vi "Multichannel Recording0.2.vi"() -> ()   [LabVIEW 2014]
uses:
  Enum State Typedef.ctl
  <vilib>/Utility/error.llb/DialogType.ctl
  <vilib>/_DAQmxBase/Internals/DAQmxBase Create Channel (AI-Voltage-Basic).vi
  <vilib>/_DAQmxBase/Internals/DAQmxBase Timing (Sample Clock).vi
  <vilib>/_DAQmxBase/Internals/DAQmxBase Read (Analog 2D DBL NChan NSamp).vi
panel:
  in  "Open Button":bool
  in  "Tab Control":T1(tab)
  in  "Use Channel 0":bool caption="In Use?"
  in  "Amplifier Channel 0":T2 {"Amplifier Model" items=["Select a Model", "AM 1700", "BMA 200"]}
  out "Channel 0 Chart":waveform(dbl)(graph)
  in  "User Data Channel 0":T3
  in  "Use Channel 1":bool caption="In Use?"
  out "Channel 1 Chart":waveform(dbl)(graph)
  in  "User Data Channel 1":T3
  in  "Amplifier Channel 1":T2 {"Amplifier Model" items=["Select a Model", "AM 1700", "BMA 200"]}
  in  "Use Channel 2":bool caption="In Use?"
  out "Channel 2 Chart":waveform(dbl)(graph)
  in  "User Data Channel 2":T3
  in  "Amplifier Channel 2":T2 {"Amplifier Model" items=["Select a Model", "AM 1700", "BMA 200"]}
  in  "Use Channel 3":bool caption="In Use?"
  out "Channel 3 Chart":waveform(dbl)(graph)
  in  "User Data Channel 3":T3
  in  "Amplifier Channel 3":T2 {"Amplifier Model" items=["Select a Model", "AM 1700", "BMA 200"]}
  out "Overview Chart":waveform(dbl)[](graph)
  in  "Stop Preview":bool
  in  "OK Button":bool
  out "State":T4
  in  "Clear Display":bool
  in  "Preview Button":bool
  out "Iterations Recorded":i32
  in  "Recording Time (seconds)":dbl
  in  "Sample Rate":i32=1000
  in  "Stop Button":bool
  out "Start Time hr/min":string
  out "Date mm/dd/yy":string
  in  "Exit Button":bool
  in  "Record Button":bool
  # "MSU EFISH Lab Multi-Channel Electronic Pulse Recorder"
  # "Must enter numbers into here before you start"
  # "Blue for On\nOrange for Off"
  # "DC"
  # "AC"
  # "Blue for AC and Orange for DC"
  # "Blue for On\nOrange for Off"
  # "DC"
  # "AC"
  # "Blue for AC and Orange for DC"
  # "Blue for On\nOrange for Off"
  # "DC"
  # "AC"
  # "Blue for AC and Orange for DC"
  # "Blue for On\nOrange for Off"
  # "DC"
  # "AC"
  # "Blue for AC and Orange for DC"
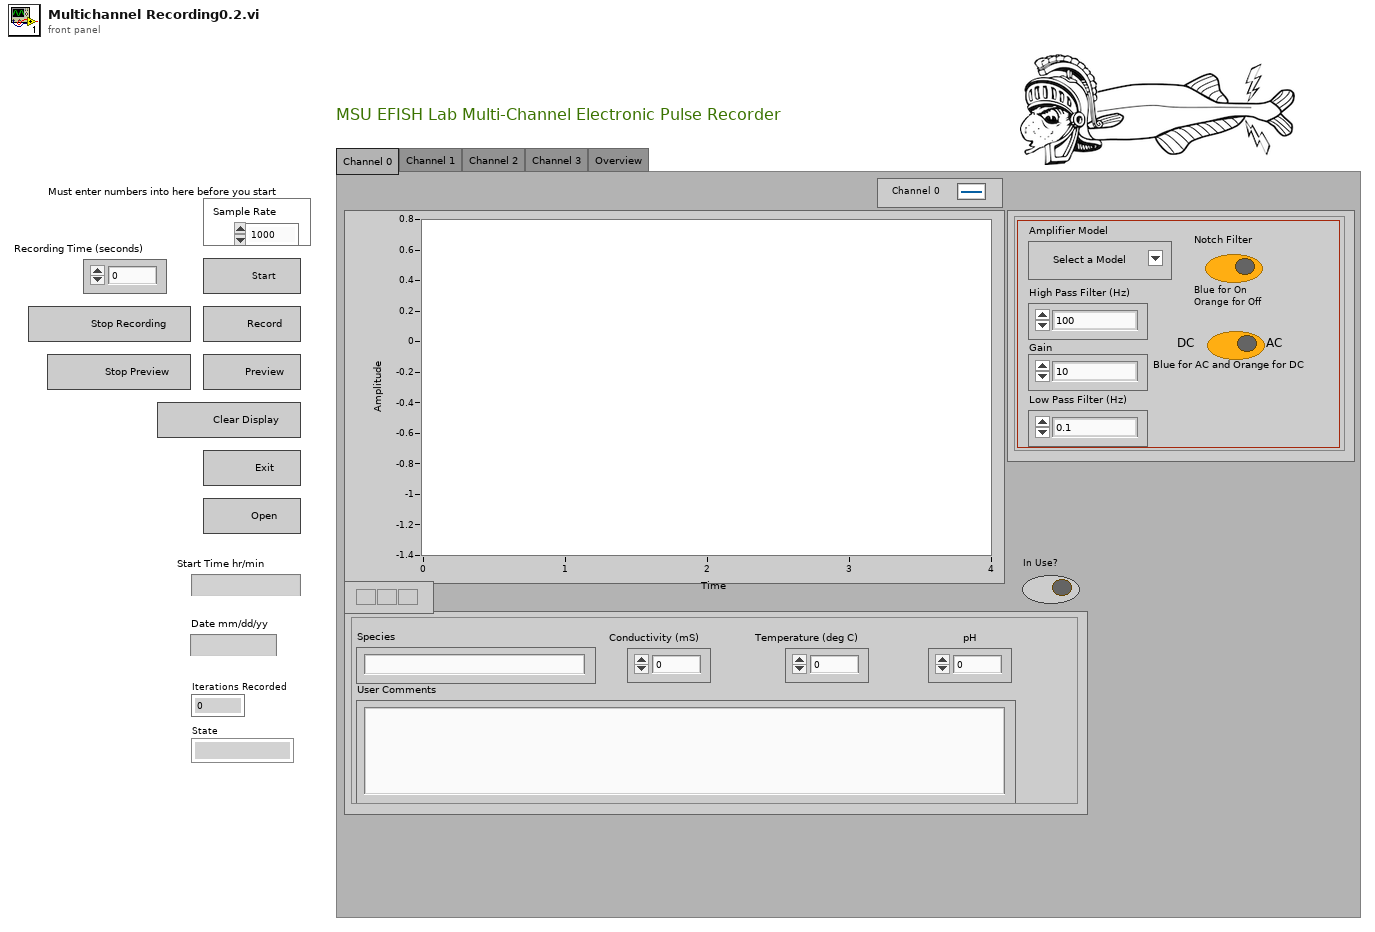
[diagram p1: front panel]
types:
  T1 = enum32{"Channel 0", "Channel 1", "Channel 2", "Channel 3", "Overview"}
  T2 = cluster{"Low Pass Filter (Hz)":enum16{"0.1", "1", "3", "10", "30", "100", "300"}, "Gain ":enum16{"10", "20", "50", "100", "200", "500", "1000", "2k", "5k", "10k", "20k", "50k"}, "High Pass Filter (Hz)":enum16{"100", "500", "1000", "3000", "5000", "10,000", "20,000", "30,000", "50,000"}, "Notch Filter":bool, "Amplifier Model":u16, "AC/DC Switch":bool}
  T3 = cluster{"pH":dbl, "Conductivity (mS)":dbl, "Temperature (deg C)":dbl, "User Comments":string, "Species":string}
  T4 = typedef "Enum State Typedef.ctl" = enum16{"", "Open FIle", "Beginning State", "Set the Sample Clock", "Prepreview Handling", "Clear Display", "Preview Data", "Stop", "Exit", "Record", "Create File"}
  T5 = enum16{"open", "open or create", "create or replace", "create", "open (read-only)"}
  T6 = cluster{"Waveform":waveform(dbl), "Waveform":waveform(dbl), "Waveform":waveform(dbl), "Waveform":waveform(dbl), waveform(dbl)[]}
  T7 = cluster{"tdms file out":refnum<k34>, "tdms file out":refnum<k34>, "tdms file out":refnum<k34>, "tdms file out":refnum<k34>}
  T8 = cluster{"Use Channel 0":bool, "Use Channel 1":bool, "Use Channel 2":bool, "Use Channel 3":bool}
  T9 = typedef "DialogType.ctl" = u16
  T10 = cluster{"data":dbl[][], dbl[][], i32, i32, dbl, "Use Channel 0":bool}
  T11 = cluster{"data":dbl[][], dbl[][], i32, i32, dbl, "Use Channel 1":bool}
  T12 = cluster{"data":dbl[][], dbl[][], i32, i32, dbl, "Use Channel 2":bool}
  T13 = cluster{"data":dbl[][], dbl[][], i32, i32, dbl, "Use Channel 3":bool}
  T14 = cluster{"Waveform":waveform(dbl), "Waveform":waveform(dbl), "Waveform":waveform(dbl), "Waveform":waveform(dbl)}
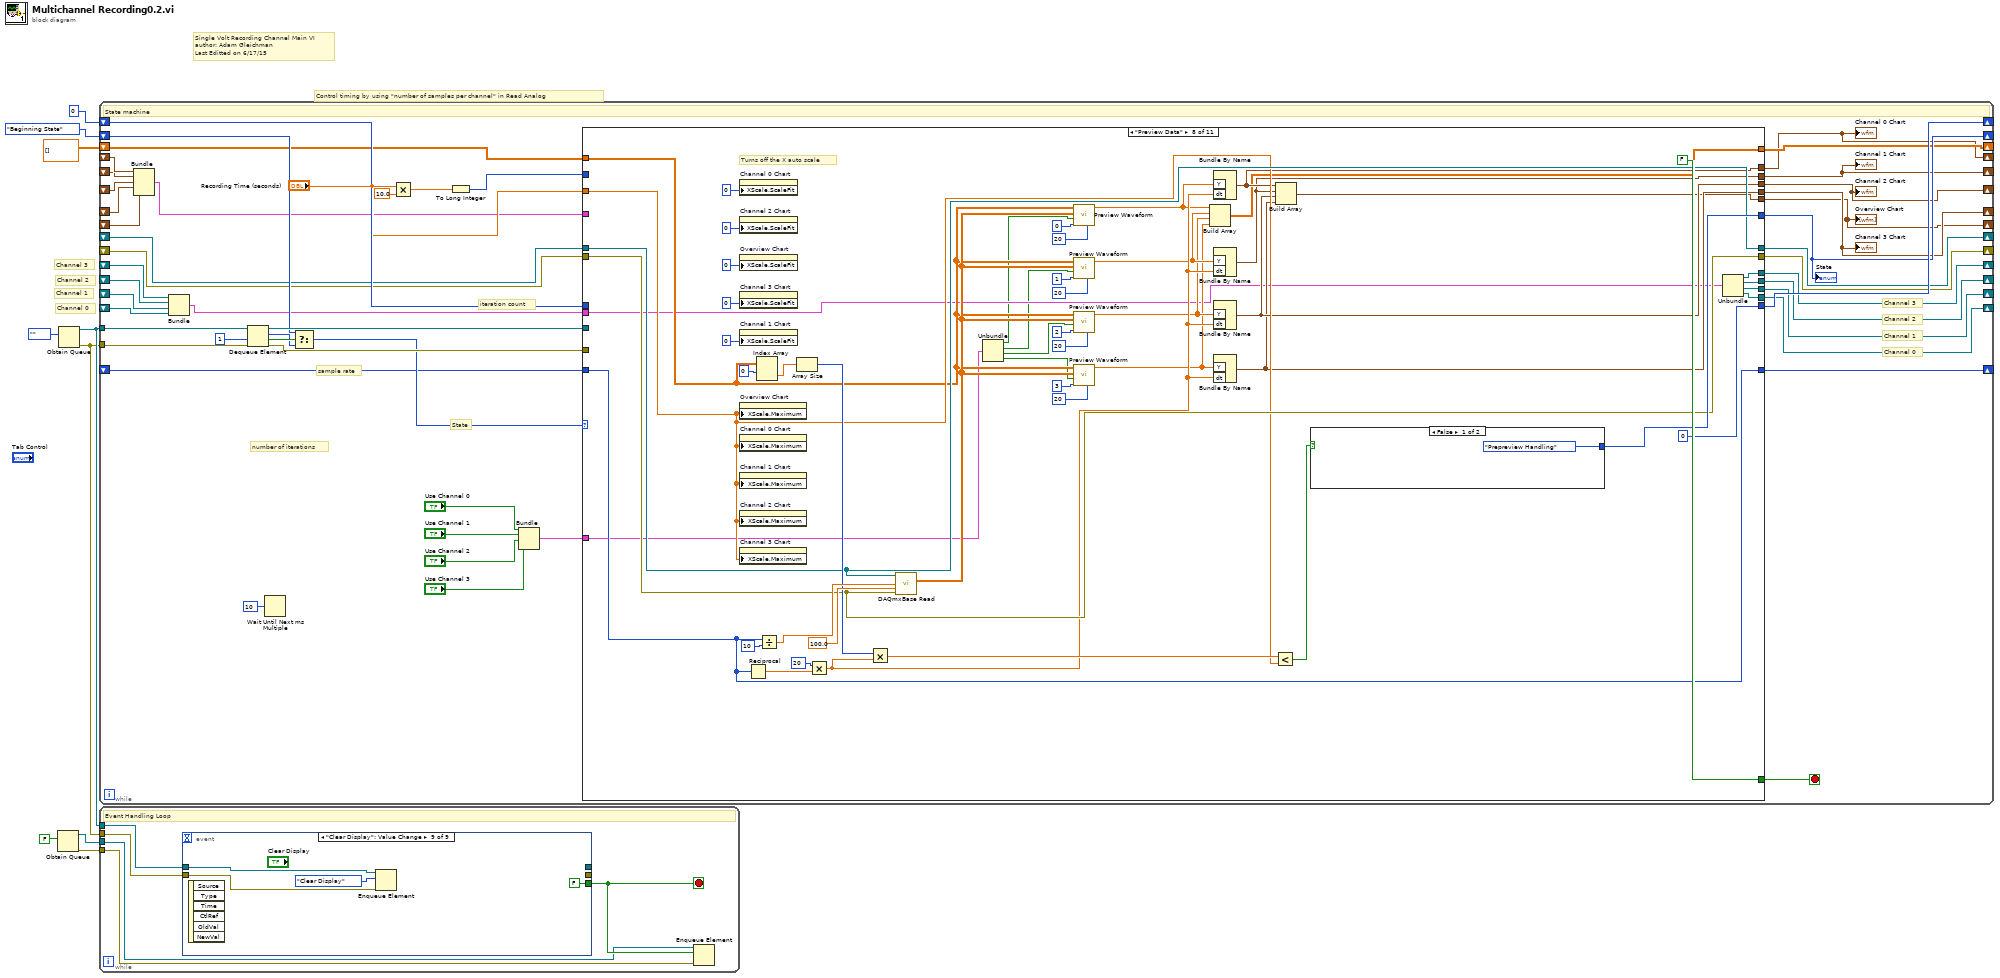
[diagram p0: block diagram]
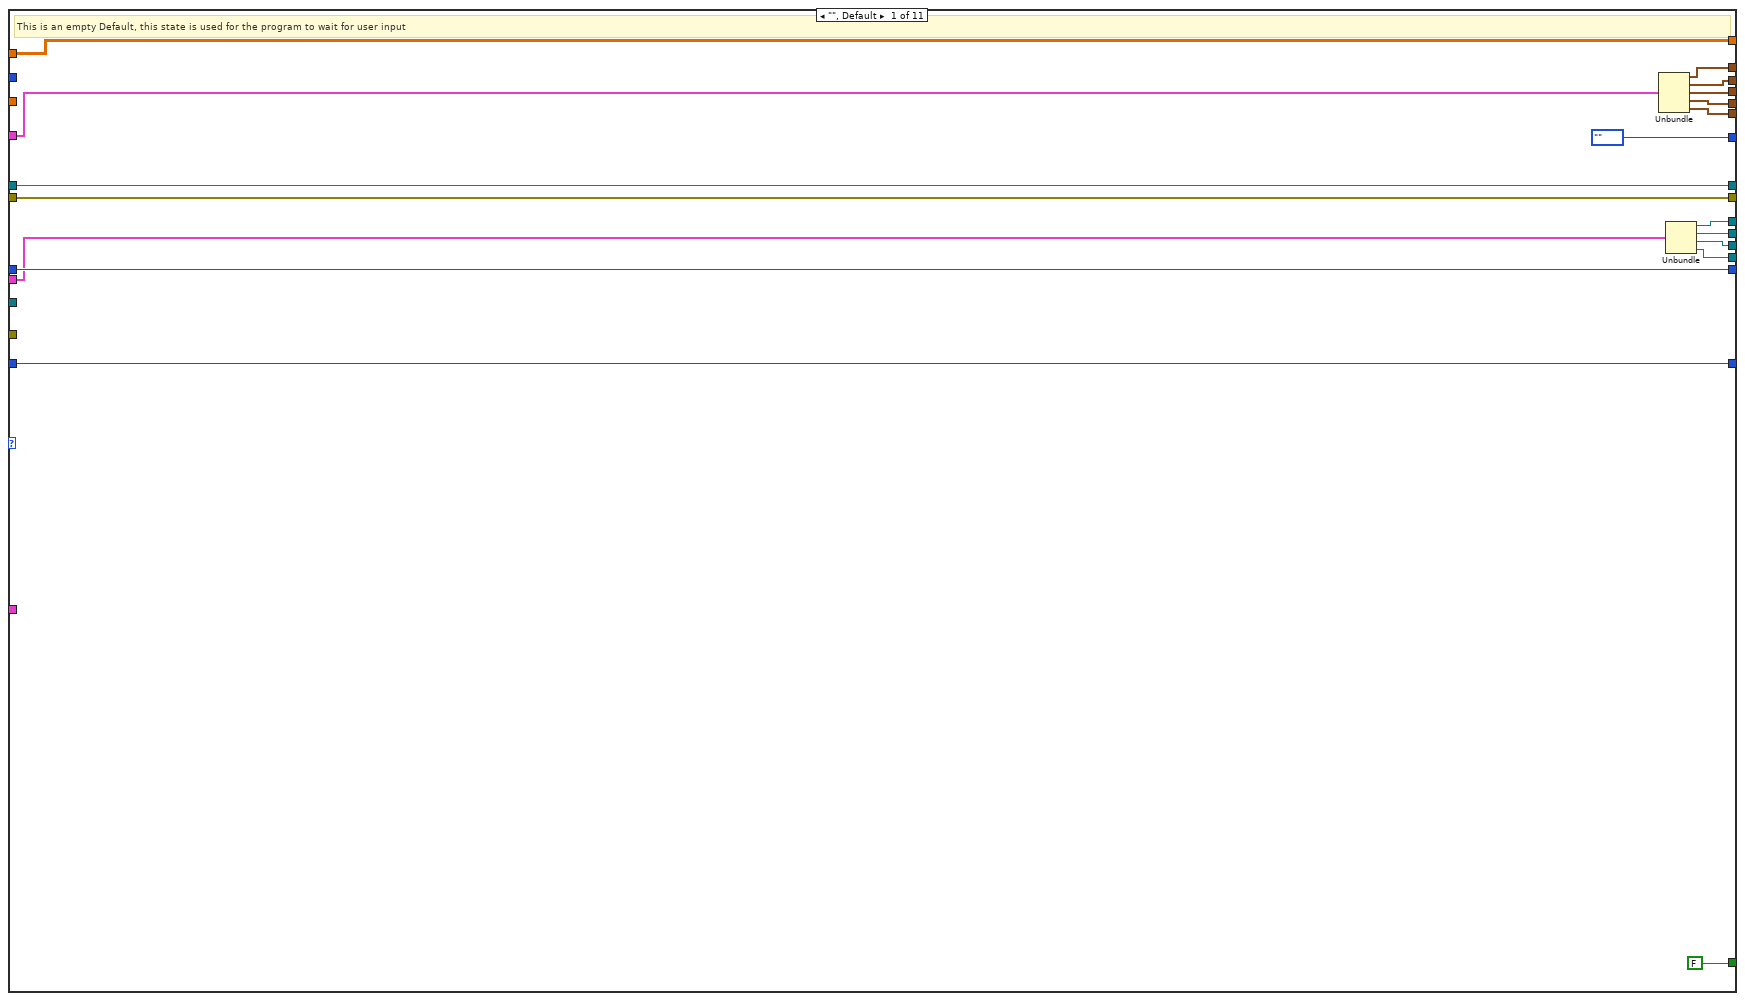
[diagram p2: hidden frame]
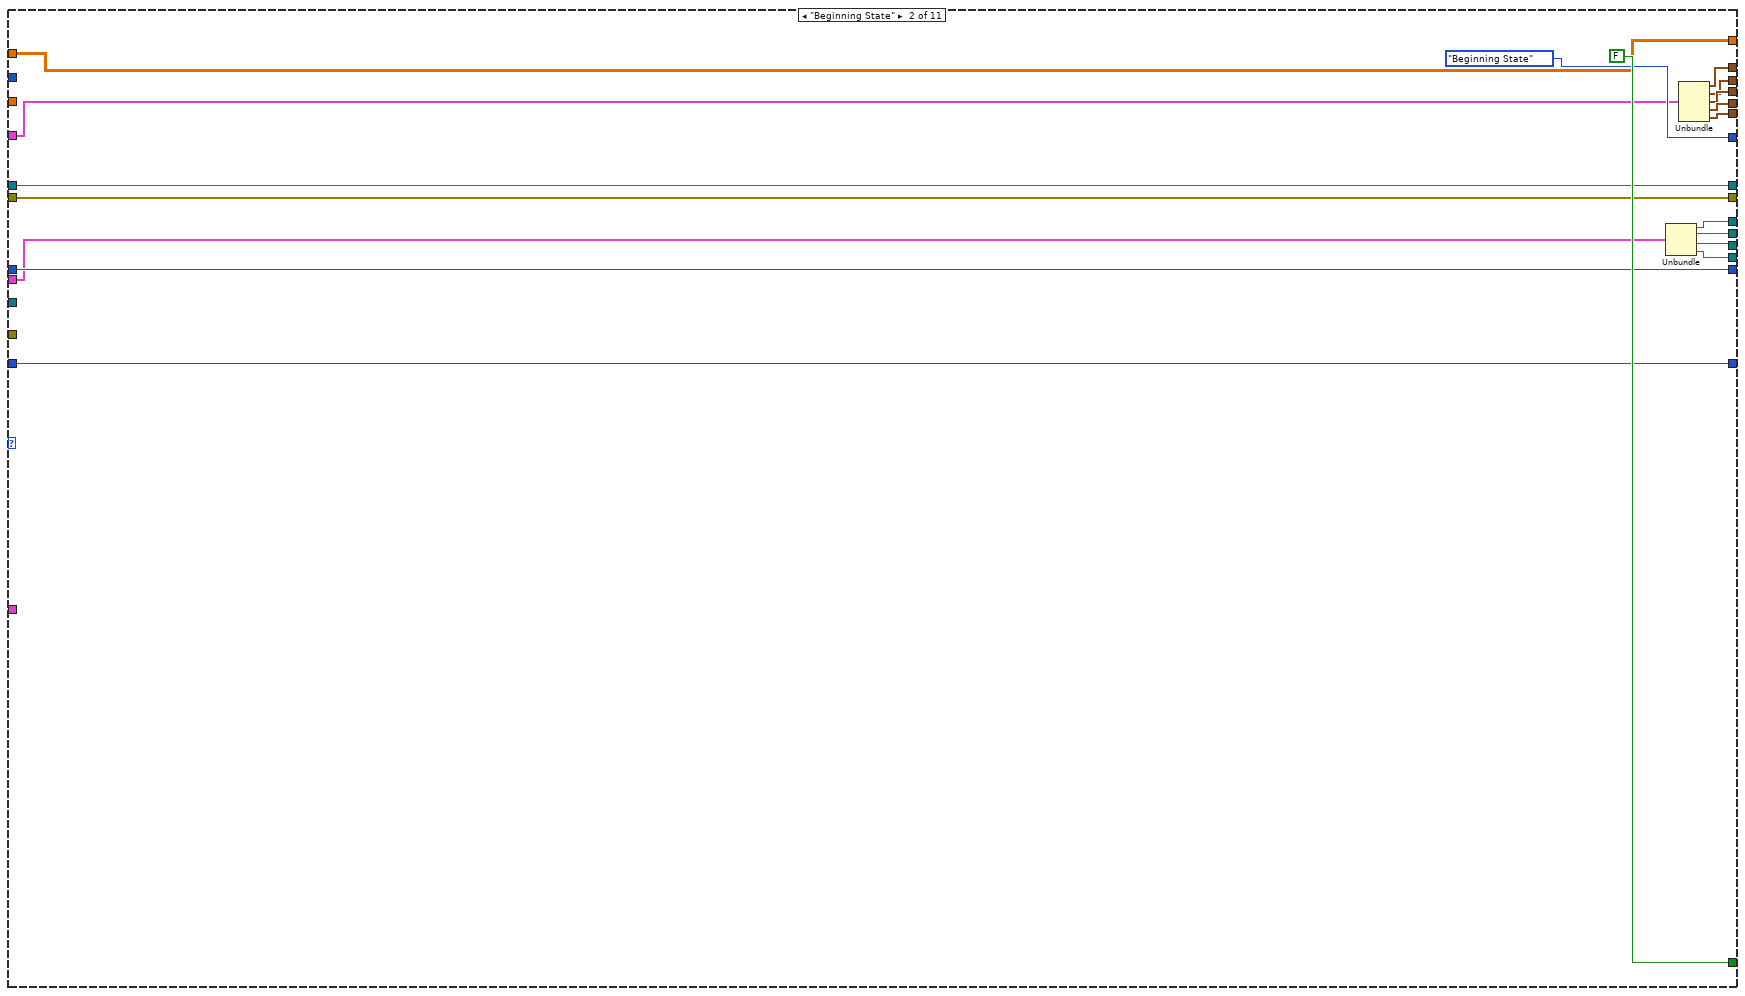
[diagram p3: hidden frame]
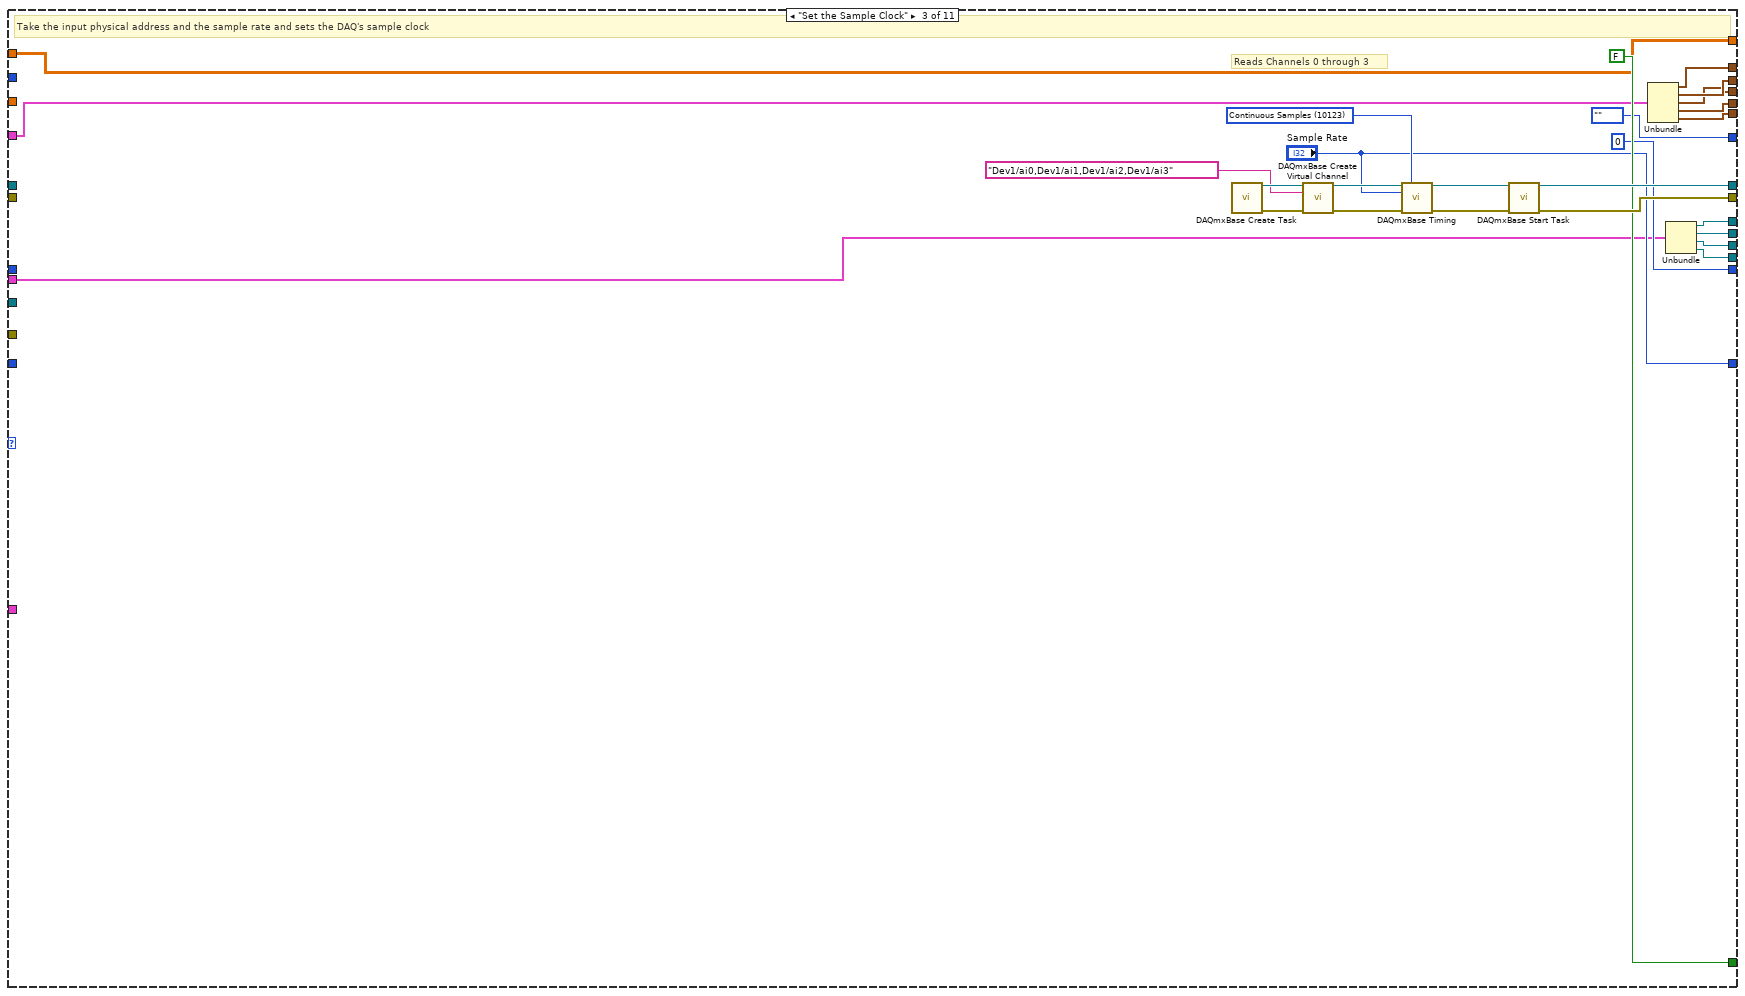
[diagram p4: hidden frame]
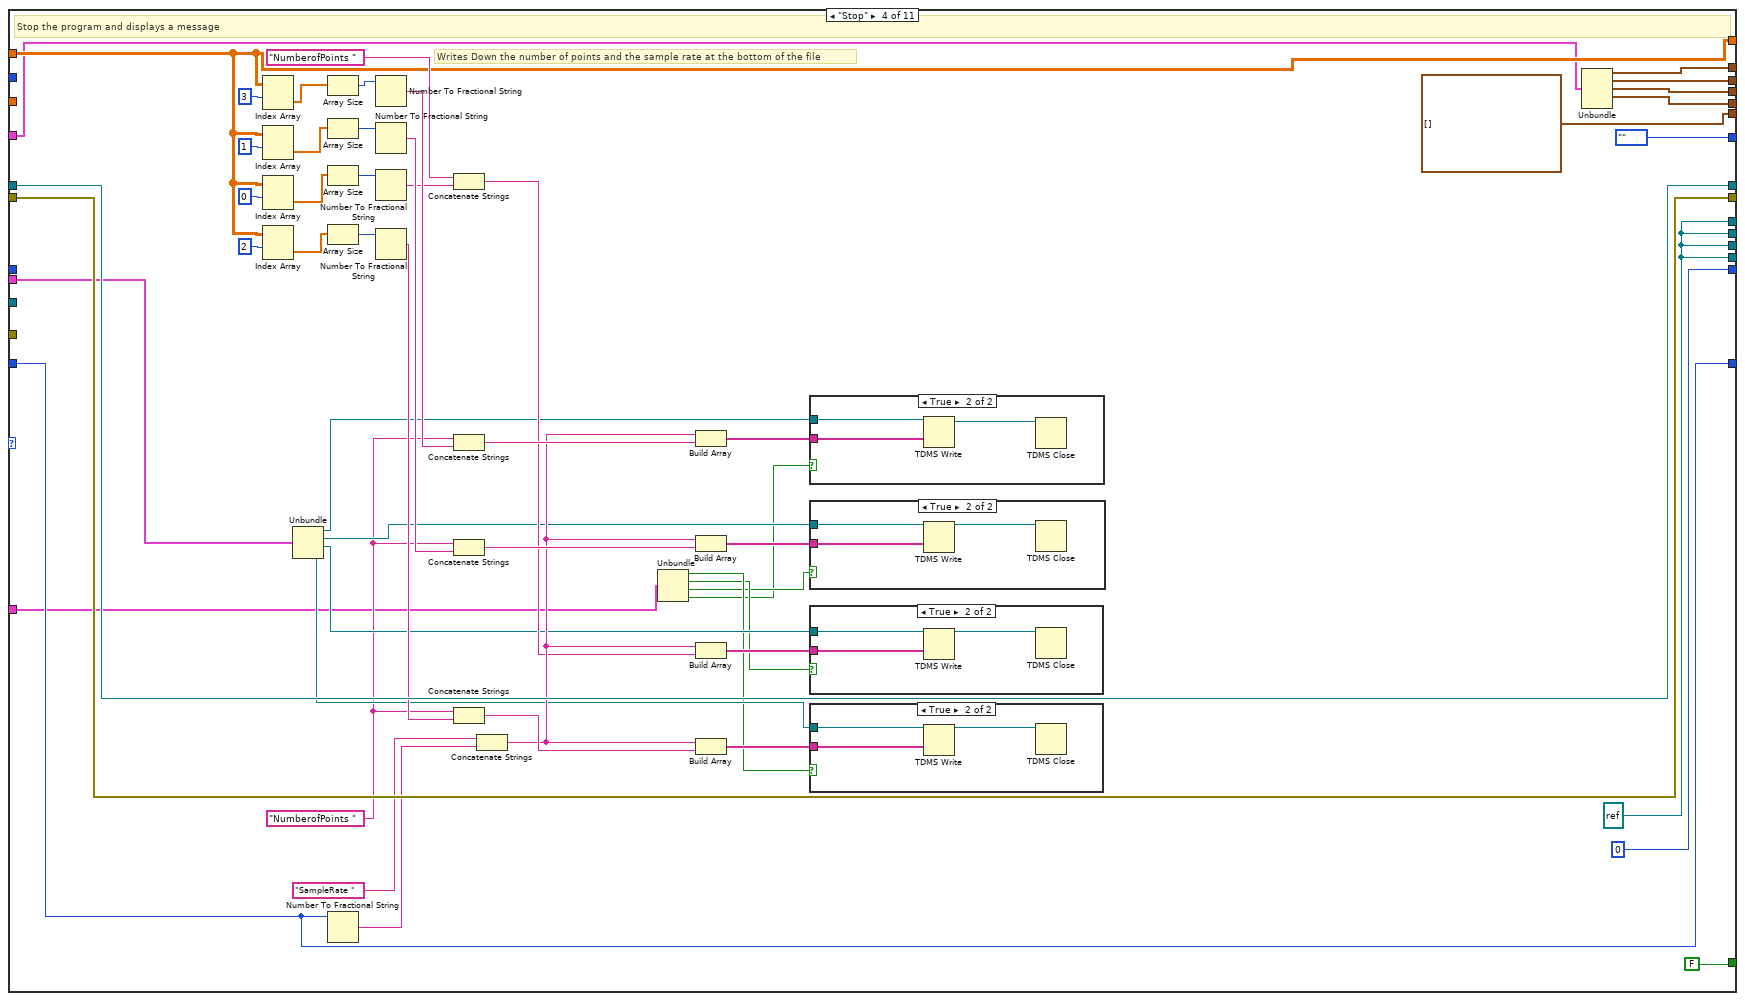
[diagram p5: hidden frame]
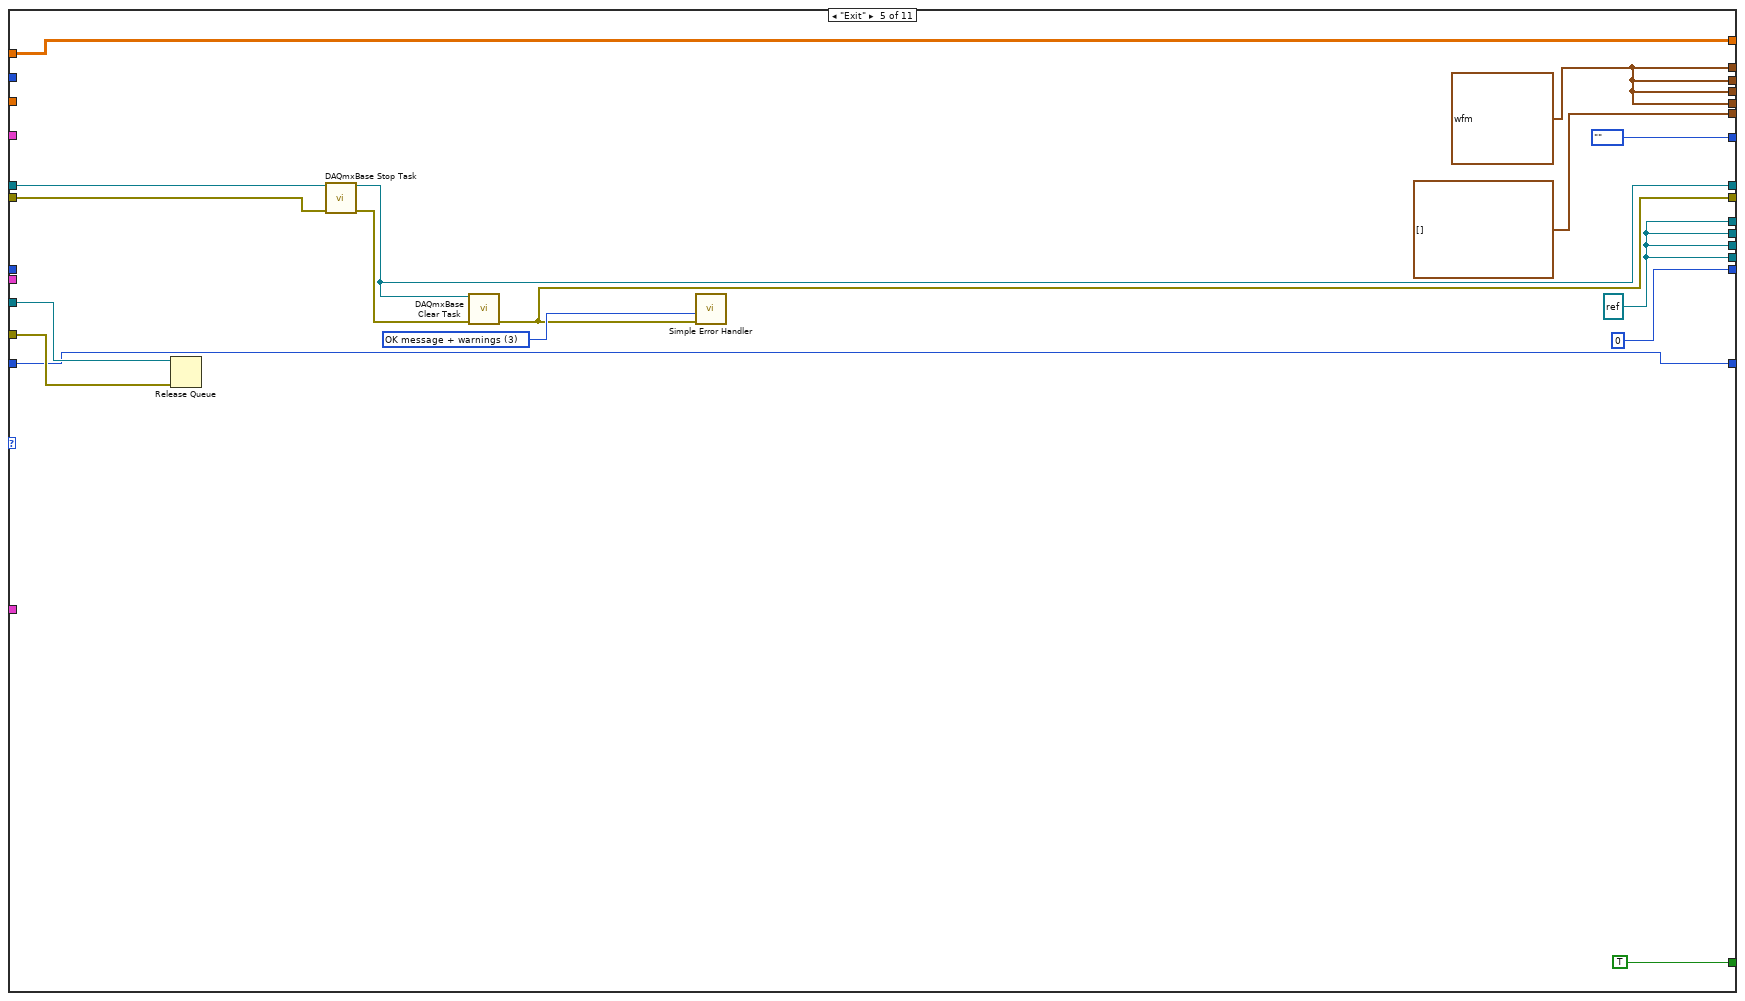
[diagram p10: hidden frame]
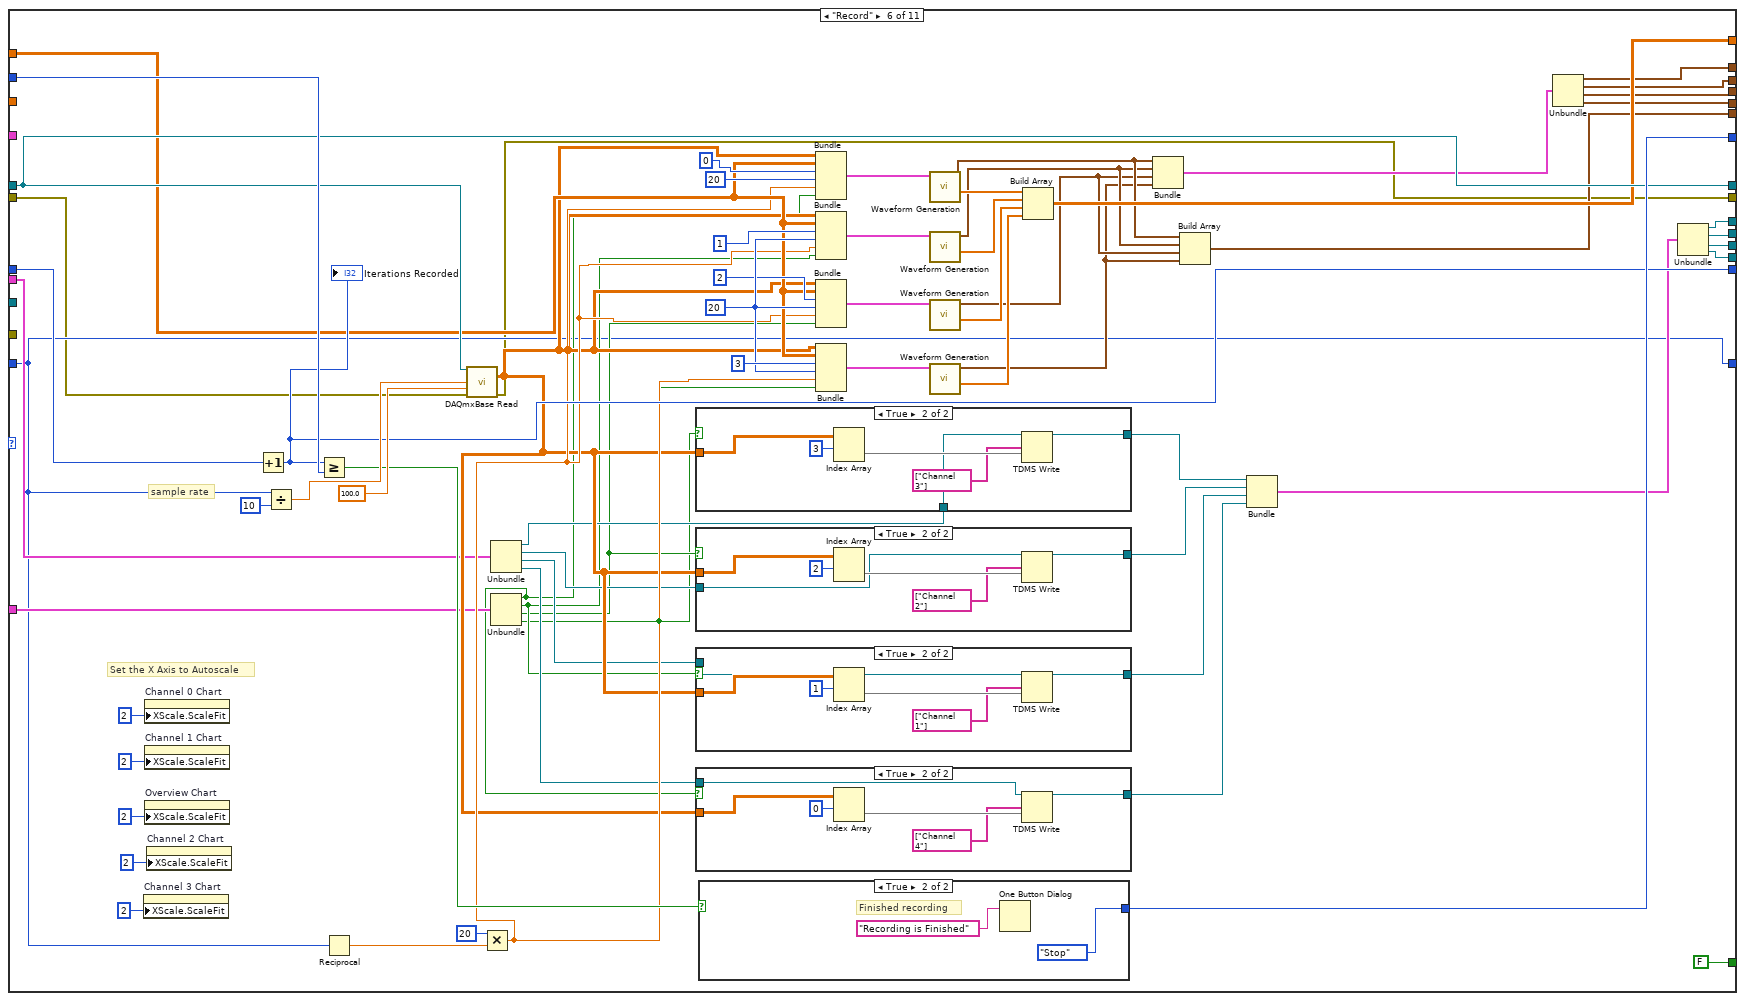
[diagram p11: hidden frame]
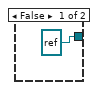
[diagram p12: hidden frame]
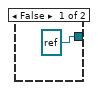
[diagram p13: hidden frame]
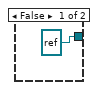
[diagram p14: hidden frame]
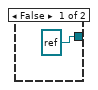
[diagram p15: hidden frame]
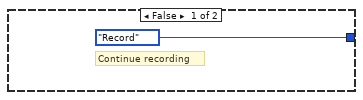
[diagram p16: hidden frame]
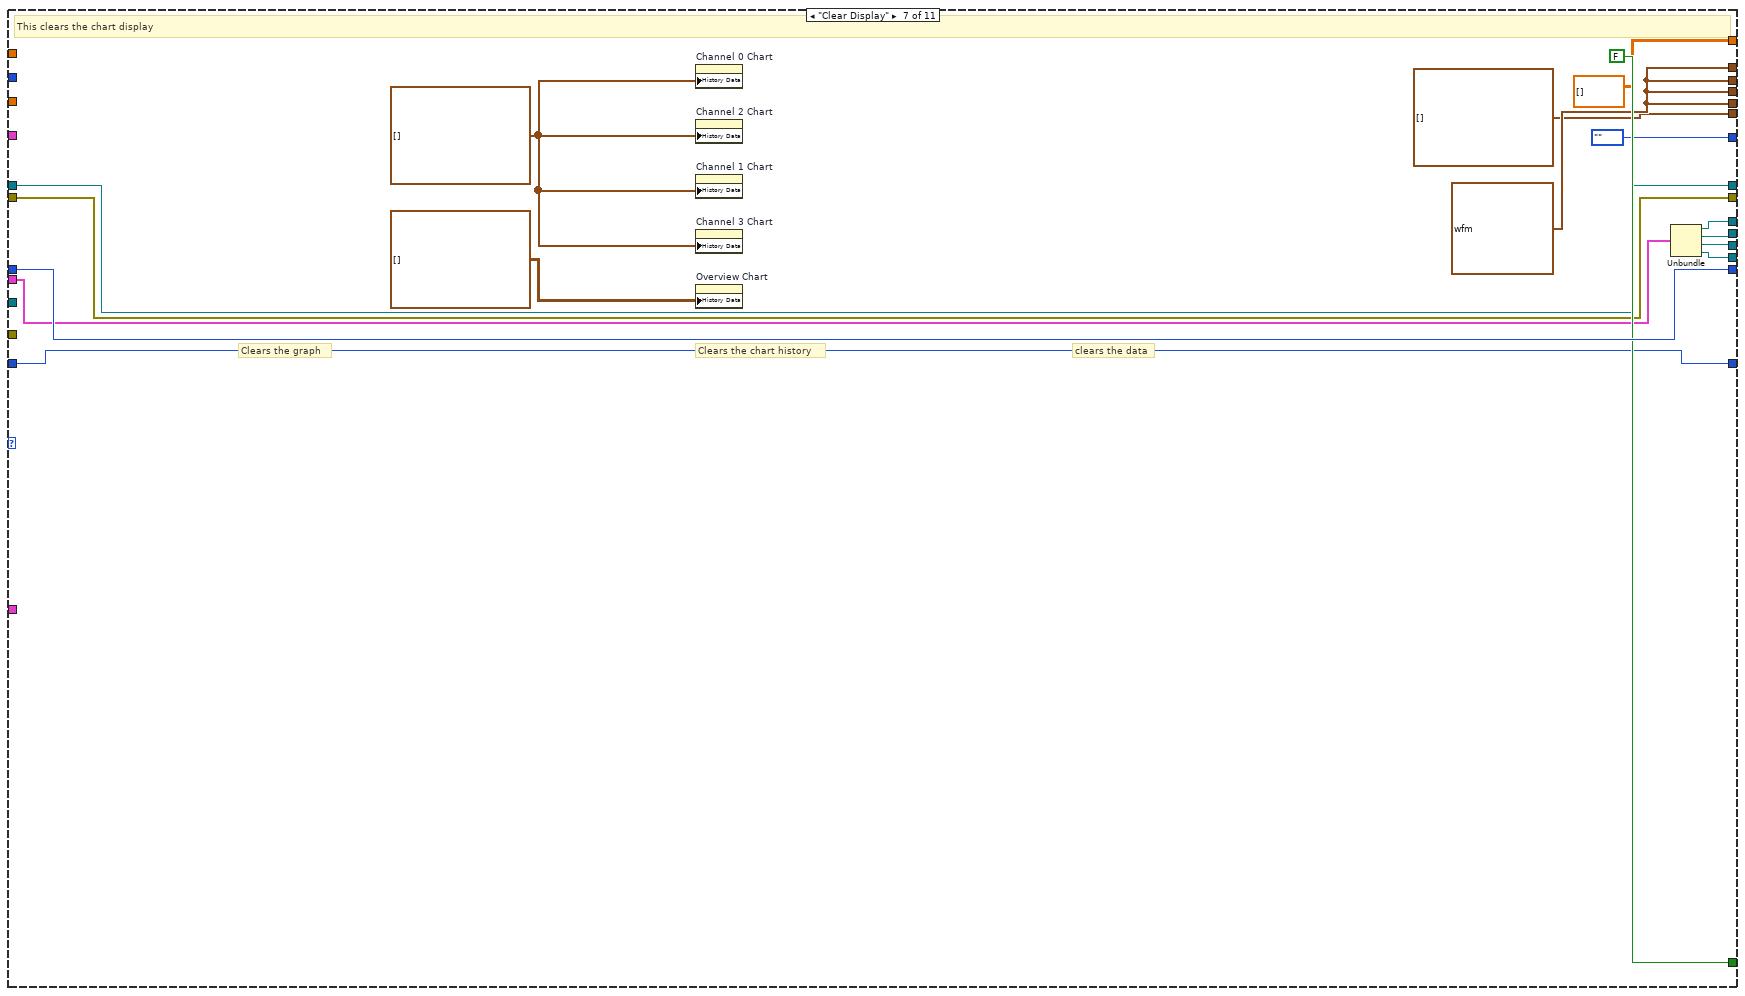
[diagram p17: hidden frame]
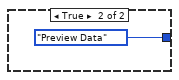
[diagram p18: hidden frame]
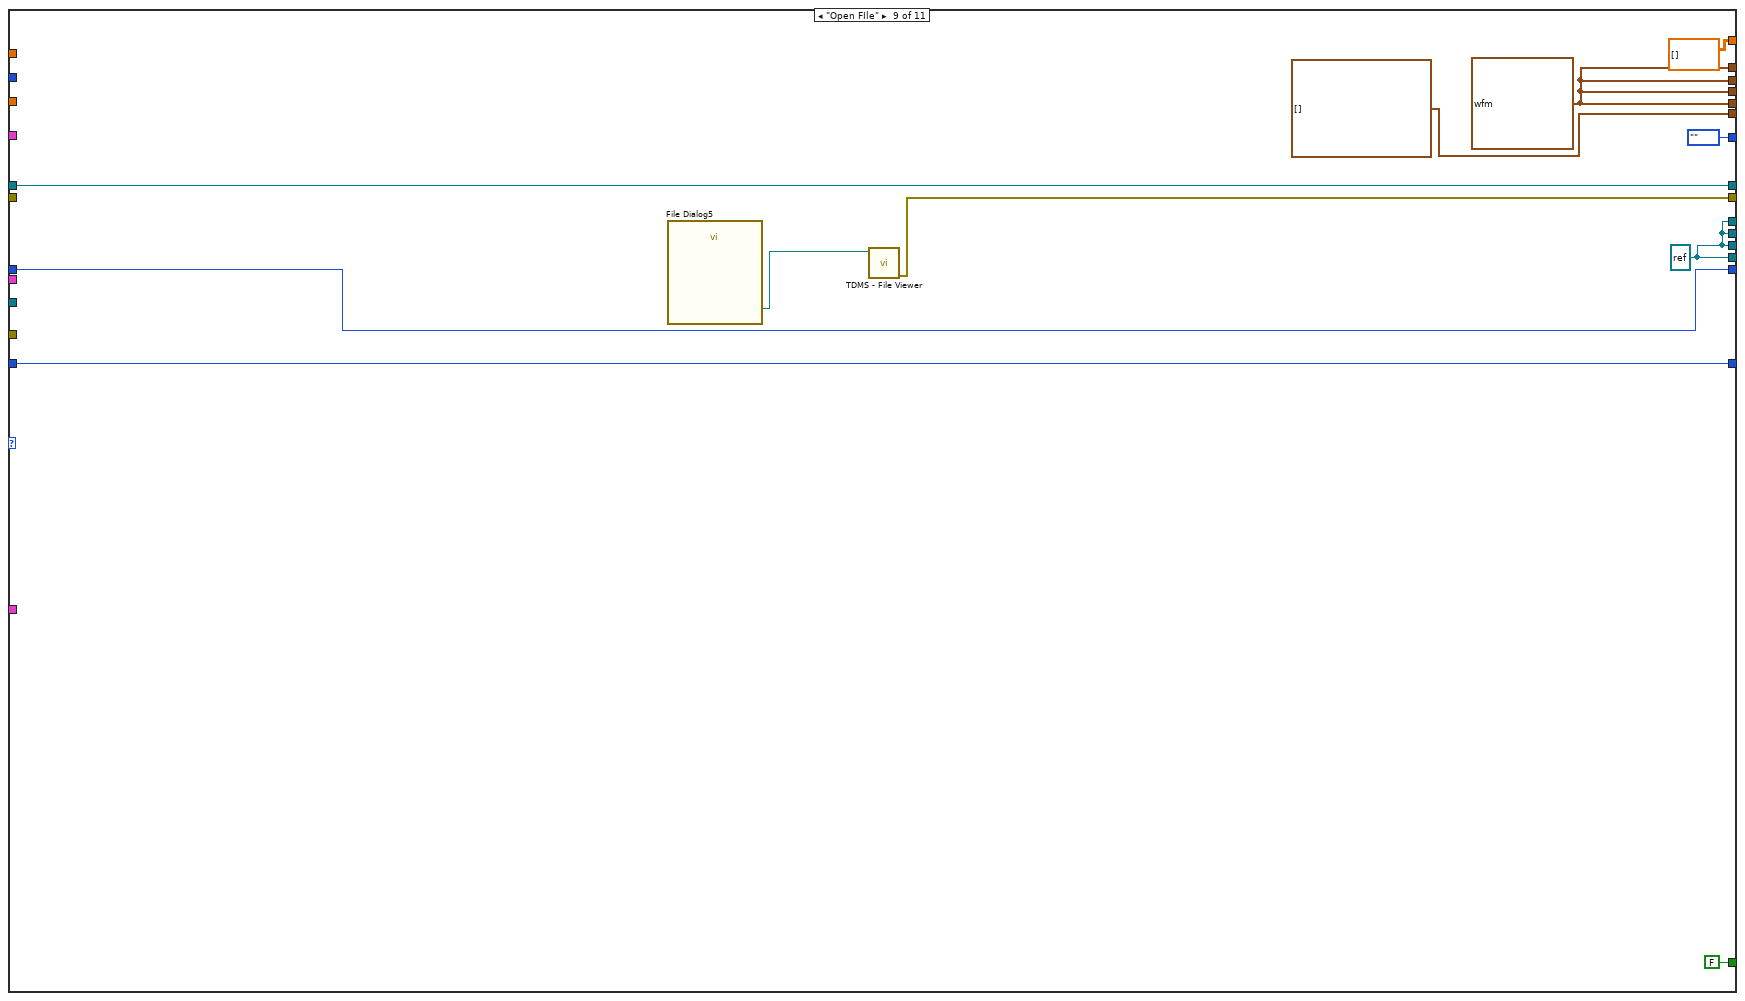
[diagram p19: hidden frame]
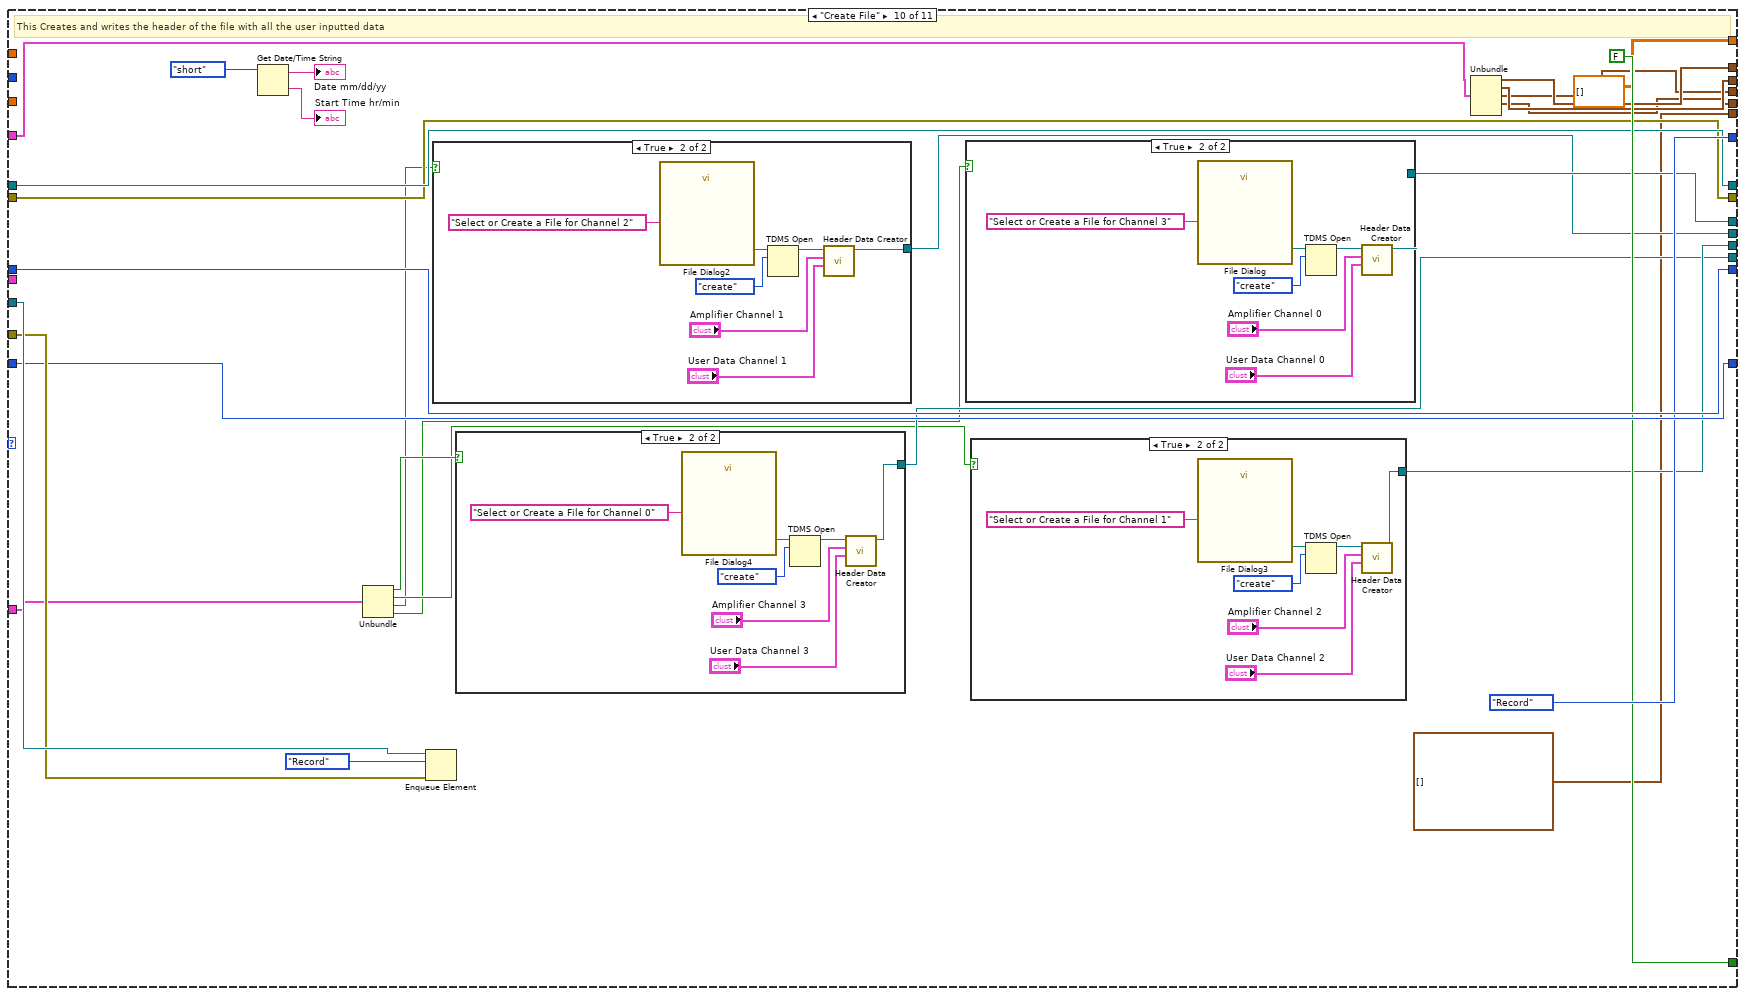
[diagram p20: hidden frame]
diagram:
  # "Channel 0"
  # "Channel 1"
  # "Channel 2"
  # "Channel 3"
  # "Single Volt Recording Channel Main VI\nauthor: Adam Gleichman\nLast Editted on 6/17/15"
  # "Control timing by using \"number of samples per channel\" in Read Analog"
  n1 = Obtain Queue(element data type=FALSE) -> (queue out=w2:refnum<queue>, error out=w1:errorcluster)  [unwired: 4 in, 1 out]
  n2 = Obtain Queue(element data type=Enum_State_Typedef."" ("State")) -> (queue out=w8:refnum<queue>, error out=w7:errorcluster)  [unwired: 4 in, 1 out]
  n3 = while {
    tunnel: w8 -> [w60]
    tunnel: w7 -> [w59]
    shift-right: [w52] -> _
    shift-left: 0 -> [w53]
    shift-right: [w47] -> _
    shift-left: Enum_State_Typedef."Beginning State" ("State") -> [w49]
    shift-right: [w45] -> _
    shift-left: _ -> [w46]
    shift-right: [w41] -> _
    shift-left: dbl[][] [] -> [w42]
    shift-right: [w31] -> _
    shift-left: _ -> [w16]
    shift-right: [w39] -> _
    shift-left: _ -> [w37]
    shift-right: [w38] -> _
    shift-left: _ -> [w36]
    shift-right: [w33] -> _
    shift-left: _ -> [w15]
    shift-right: [w32] -> _
    shift-left: _ -> [w17]
    shift-right: [w34] -> _
    shift-left: _ -> [w18]
    shift-right: [w30] -> _
    shift-left: _ -> [w23]
    shift-right: [w29] -> _
    shift-left: _ -> [w22]
    shift-right: [w27] -> _
    shift-left: _ -> [w21]
    shift-right: [w28] -> _
    shift-left: _ -> [w20]
    shift-right: [w26] -> _
    shift-left: _ -> [w25]
    stop <- w58 stop-if-true
    # "Channel 0"
    # "Channel 1"
    # "Channel 2"
    # "Channel 3"
    # "State"
    # "iteration count"
    # "sample rate"
    # "number of iterations"
    # "State machine"
    n4 = Bundle("Waveform"=w18, "Waveform"=w17, "Waveform"=w16, "Waveform"=w15, w25) -> (w24:T6)  [unwired: 1 in]
    n5 = Bundle("tdms file out"=w23, "tdms file out"=w22, "tdms file out"=w21, "tdms file out"=w20) -> (w19:T7)  [unwired: 1 in]
    n6 = Dequeue Element(queue=w60, timeout in ms (-1)=1, error in (no error)=w59) -> (queue out=w57:refnum<queue>, element=w50:T4, timed out?=w51:bool, error out=w56:errorcluster)
    n7 = Wait Until Next ms Multiple(millisecond multiple=u32 10) -> ()  [unwired: 1 out]
    n8 = Select(t=w49, s=w51, f=w50) -> (s? t:f=w48:T4)
    n9 = Multiply(x="Recording Time (seconds)", y=10.0) -> (x*y=w35:dbl)
    n10 = To Long Integer(number=w35) -> (32bit integer=w54:i32)
    n11 = Bundle("Use Channel 0"="Use Channel 0", "Use Channel 1"="Use Channel 1", "Use Channel 2"="Use Channel 2", "Use Channel 3"="Use Channel 3") -> (w10:T8)  [unwired: 1 in]
    n12 = case shown="\"Preview Data\"" w48 {
      tunnel: [FALSE FALSE FALSE FALSE TRUE FALSE FALSE FALSE FALSE FALSE FALSE] -> w58
      tunnel: w57 -> [_ _ _ _ w198 _ _ _ _ w411 _]
      tunnel: w56 -> [_ _ _ _ w197 _ _ _ _ w410 _]
      tunnel: w37 -> [w74 w94 _ w172 w201 w259 w314 w359 w378 w404 w455]
      tunnel: w36 -> [w73 w95 _ w171 w200 w205 w313 w358 _ w403 w454]
      tunnel: w46 -> [w75 w92 _ w169 w194 w206 w312 w355 w376 w407 w456]
      tunnel: w54 -> [_ _ _ _ _ w267 _ _ _ _ _]
      tunnel: w53 -> [w77 w91 _ _ _ w268 w317 _ w377 w408 w457]
      tunnel: [w77 w91 0 ("Sample Rate") 0 0 w262 w317 0 w377 w408 w457] -> w52
      tunnel: [Enum_State_Typedef."" ("State") Enum_State_Typedef."Beginning State" ("State") Enum_State_Typedef."" ("State") Enum_State_Typedef."" ("State") Enum_State_Typedef."" ("State") w264 Enum_State_Typedef."" ("State") w363 Enum_State_Typedef."" ("State") Enum_State_Typedef."Record" ("State") Enum_State_Typedef."Preview Data" ("State")] -> w47
      tunnel: [w75 w92 "Sample Rate" w169 w194 w206 w312 w355 w376 w407 w456] -> w45
      tunnel: [w72 w90 w108 w151 w193 w240 dbl[][] [] w328 dbl[][] [] dbl[][] [] dbl[][] []] -> w41
      tunnel: w42 -> [w72 w90 w108 w151 w193 w247 _ w338 _ _ _]
      tunnel: "Recording Time (seconds)" -> [_ _ _ _ _ _ _ w339 _ _ _]
      tunnel: [w74 w94 w115 w172 w192 w259 w314 w359 w378 w404 w455] -> w39
      tunnel: [w73 w95 w114 w171 w191 w204 w313 w358 w379 w403 w454] -> w38
      tunnel: [w68 w86 w104 w143 w189 w231 w309 w335 w382 w390 w452] -> w31
      tunnel: [w69 w85 w105 w144 w189 w232 w309 w336 w382 w391 w452] -> w32
      tunnel: [w67 w87 w103 w142 w189 w230 w309 w334 w382 w389 w452] -> w33
      tunnel: [w70 w84 w106 w145 w189 w233 w309 w337 w382 w392 w452] -> w34
      tunnel: [w64 w82 w100 w167 w190 w210 w305 w326 w381 w398 w447] -> w30
      tunnel: [w63 w81 w99 w167 w190 w209 w304 w325 w381 w397 w446] -> w29
      tunnel: [w62 w80 w98 w167 w190 w208 w303 w324 w381 w396 w445] -> w27
      tunnel: [w61 w79 w97 w167 w190 w207 w302 w323 w381 w395 w444] -> w28
      tunnel: [w66 w88 w102 waveform(dbl)[] [] waveform(dbl)[] [] w225 waveform(dbl)[] [] w333 waveform(dbl)[] [] waveform(dbl)[] [] waveform(dbl)[] []] -> w26
      tunnel: w24 -> [w71 w89 w107 w146 _ _ _ _ _ w393 _]
      tunnel: w19 -> [w65 w83 w101 w141 _ w239 w306 w327 _ _ w448]
      tunnel: w10 -> [_ _ _ w135 _ w224 _ w322 _ w388 _]
      frame "", Default {
        # "This is an empty Default, this state is used for the program to wait for user input"
        n13 = Unbundle(w71) -> ("Waveform"=w70:waveform(dbl), "Waveform"=w69:waveform(dbl), "Waveform"=w68:waveform(dbl), "Waveform"=w67:waveform(dbl), w66:waveform(dbl)[])
        n14 = Unbundle(w65) -> ("tdms file out"=w64:refnum<k34>, "tdms file out"=w63:refnum<k34>, "tdms file out"=w62:refnum<k34>, "tdms file out"=w61:refnum<k34>)
      }
      frame "Beginning State" {
        n15 = Unbundle(w83) -> ("tdms file out"=w82:refnum<k34>, "tdms file out"=w81:refnum<k34>, "tdms file out"=w80:refnum<k34>, "tdms file out"=w79:refnum<k34>)
        n16 = Unbundle(w89) -> ("Waveform"=w84:waveform(dbl), "Waveform"=w85:waveform(dbl), "Waveform"=w86:waveform(dbl), "Waveform"=w87:waveform(dbl), w88:waveform(dbl)[])
      }
      frame "Set the Sample Clock" {
        w118 = 10123 items=["Finite Samples"=10178, "Continuous Samples"=10123, "Hardware Timed Single Point"=12522] ("sample mode")
        # "Reads Channels 0 through 3"
        # "Take the input physical address and the sample rate and sets the DAQ's sample clock"
        n17 = call <vilib>:"DAQmxBase Create Task.vi"() -> ("task out"=w122:refnum<k21>, "error out"=w121:errorcluster)  [unwired: 14 in]
        n18 = call-poly <vilib>:"DAQmxBase Create Virtual Channel.vi"("task in"=w122, "physical channels"=tag "Dev1/ai0,Dev1/ai1,Dev1/ai2,Dev1/ai3", "error in"=w121) -> ("task out"=w120:refnum<k21>, "error out"=w119:errorcluster)  [unwired: 11 in]
        n19 = call-poly <vilib>:"DAQmxBase Timing.vi"("task/channels in"=w120, "sample mode"=w118, "rate"="Sample Rate", "error in"=w119) -> ("task out"=w117:refnum<k21>, "error out"=w116:errorcluster)  [unwired: 10 in]
        n20 = call <vilib>:"DAQmxBase Start Task.vi"("task/channels in"=w117, "error in"=w116) -> ("task out"=w115:refnum<k21>, "error out"=w114:errorcluster)  [unwired: 12 in]
        n21 = Unbundle(w107) -> ("Waveform"=w106:waveform(dbl), "Waveform"=w105:waveform(dbl), "Waveform"=w104:waveform(dbl), "Waveform"=w103:waveform(dbl), w102:waveform(dbl)[])
        n22 = Unbundle(w101) -> ("tdms file out"=w100:refnum<k34>, "tdms file out"=w99:refnum<k34>, "tdms file out"=w98:refnum<k34>, "tdms file out"=w97:refnum<k34>)
      }
      frame "Stop" {
        w136 = "NumberofPoints " ("string")
        w167 = refnum<k34> refnum ("tdms file out")
        # "Writes Down the number of points and the sample rate at the bottom of the file"
        # "Stop the program and displays a message"
        n23 = Index Array(array=w151, index (row)=3) -> (element=w130:dbl[])  [unwired: 1 in]
        n24 = Index Array(array=w151, index (row)=1) -> (element=w128:dbl[])  [unwired: 1 in]
        n25 = Index Array(array=w151, index (row)=0) -> (element=w125:dbl[])  [unwired: 1 in]
        n26 = Index Array(array=w151, index (row)=2) -> (element=w123:dbl[])  [unwired: 1 in]
        n27 = Unbundle(w141) -> ("tdms file out"=w140:refnum<k34>, "tdms file out"=w139:refnum<k34>, "tdms file out"=w138:refnum<k34>, "tdms file out"=w137:refnum<k34>)
        n28 = Array Size(array=w130) -> (size(s)=w129:i32)
        n29 = Array Size(array=w128) -> (size(s)=w127:i32)
        n30 = Array Size(array=w125) -> (size(s)=w126:i32)
        n31 = Array Size(array=w123) -> (size(s)=w124:i32)
        n32 = Number To Fractional String(number=w169) -> (F-format string=w168:string)  [unwired: 3 in]
        n33 = Number To Fractional String(number=w129) -> (F-format string=w165:string)  [unwired: 3 in]
        n34 = Number To Fractional String(number=w127) -> (F-format string=w157:string)  [unwired: 3 in]
        n35 = Number To Fractional String(number=w126) -> (F-format string=w152:string)  [unwired: 3 in]
        n36 = Number To Fractional String(number=w124) -> (F-format string=w161:string)  [unwired: 3 in]
        n37 = Concatenate Strings("NumberofPoints " ("string"), w152) -> (w149:string)
        n38 = Concatenate Strings(w136, w165) -> (w164:string)
        n39 = Concatenate Strings(w136, w157) -> (w156:string)
        n40 = Concatenate Strings(w136, w161) -> (w160:string)
        n41 = Concatenate Strings("SampleRate ", w168) -> (w150:string)
        n42 = Unbundle(w135) -> ("Use Channel 0"=w134:bool, "Use Channel 1"=w133:bool, "Use Channel 2"=w132:bool, "Use Channel 3"=w131:bool)
        n43 = Build Array(w150, w164) -> (w163:string[])
        n44 = Build Array(w150, w156) -> (w155:string[])
        n45 = Build Array(w150, w149) -> (w148:string[])
        n46 = Build Array(w150, w160) -> (w159:string[])
        n47 = case shown="True" w131 {
          tunnel: w163 -> [_ w187]
          tunnel: w140 -> [_ w186]
          frame False {
          }
          frame True {
            n48 = TDMS Write(0:w186, 9:w187) -> (4:w185:refnum<k34>)  [unwired: 4 in, 3 out]
            n49 = TDMS Close(11:w185) -> ()  [unwired: 1 in, 2 out]
          }
        }
        n50 = case shown="True" w132 {
          tunnel: w155 -> [_ w181]
          tunnel: w139 -> [_ w180]
          frame False {
          }
          frame True {
            n51 = TDMS Write(0:w180, 9:w181) -> (4:w179:refnum<k34>)  [unwired: 4 in, 3 out]
            n52 = TDMS Close(11:w179) -> ()  [unwired: 1 in, 2 out]
          }
        }
        n53 = case shown="True" w133 {
          tunnel: w148 -> [_ w178]
          tunnel: w138 -> [_ w177]
          frame False {
          }
          frame True {
            n54 = TDMS Write(0:w177, 9:w178) -> (4:w176:refnum<k34>)  [unwired: 4 in, 3 out]
            n55 = TDMS Close(11:w176) -> ()  [unwired: 1 in, 2 out]
          }
        }
        n56 = case shown="True" w134 {
          tunnel: w159 -> [_ w184]
          tunnel: w137 -> [_ w183]
          frame False {
          }
          frame True {
            n57 = TDMS Write(0:w183, 9:w184) -> (4:w182:refnum<k34>)  [unwired: 4 in, 3 out]
            n58 = TDMS Close(11:w182) -> ()  [unwired: 1 in, 2 out]
          }
        }
        n59 = Unbundle(w146) -> ("Waveform"=w145:waveform(dbl), "Waveform"=w144:waveform(dbl), "Waveform"=w143:waveform(dbl), "Waveform"=w142:waveform(dbl))  [unwired: 1 out]
      }
      frame "Exit" {
        w189 = waveform(dbl) {"t0"=timestamp(0 s since 1904-01-01), "dt"=1.0, "Y"=[]} ("Waveform")
        w190 = refnum<k34> refnum ("tdms file out")
        w199 = T9 3 items=["no dialog", "OK message", "continue or stop message", "OK message + warnings", "continue/stop + warnings"] ("type of dialog (OK msg:1)")
        n60 = Release Queue(queue=w198, error in (no error)=w197) -> ()  [unwired: 1 in, 3 out]
        n61 = call <vilib>:"DAQmxBase Stop Task.vi"("task/channels in"=w201, "error in"=w200) -> ("task out"=w192:refnum<k21>, "error out"=w202:errorcluster)  [unwired: 12 in]
        n62 = call <vilib>:"DAQmxBase Clear Task.vi"("task in"=w192, "error in"=w202) -> ("error out"=w191:errorcluster)  [unwired: 13 in]
        n63 = call <vilib>:"Simple Error Handler.vi"("type of dialog (OK msg:1)"=w199, "error in (no error)"=w191) -> ()  [unwired: 3 in, 5 out]
      }
      frame "Record" {
        w253 = 20
        # "sample rate"
        # "Set the X Axis to Autoscale"
        n64 = property on="Channel 3 Chart" class="WFChart (strict)"("XScale.ScaleFit"=u8 2 ("X Scale.Scale Fit")) -> ()  [unwired: 2 in, 2 out]
        n65 = property on="Channel 0 Chart" class="WFChart (strict)"("XScale.ScaleFit"=u8 2 ("X Scale.Scale Fit")) -> ()  [unwired: 2 in, 2 out]
        n66 = property on="Channel 1 Chart" class="WFChart (strict)"("XScale.ScaleFit"=u8 2 ("X Scale.Scale Fit")) -> ()  [unwired: 2 in, 2 out]
        n67 = property on="Overview Chart" class="WFChart (strict)"("XScale.ScaleFit"=u8 2 ("X Scale.Scale Fit")) -> ()  [unwired: 2 in, 2 out]
        n68 = property on="Channel 2 Chart" class="WFChart (strict)"("XScale.ScaleFit"=u8 2 ("X Scale.Scale Fit")) -> ()  [unwired: 2 in, 2 out]
        n69 = Increment(x=w268) -> (x+1=w262:i32)
        "Iterations Recorded" <- w262
        n70 = Divide(x=w206, y=10) -> (x/y=w265:dbl)
        n71 = Greater Or Equal?(x=w262, y=w267) -> (x >= y?=w263:bool)
        n72 = Reciprocal(x=w206) -> (1/x=w261:dbl)
        n73 = call-poly <vilib>:"DAQmxBase Read.vi"("task/channels in"=w259, "number of samples per channel"=w265, "timeout"=100.0, "error in"=w205) -> ("data"=w245:dbl[][], "error out"=w204:errorcluster)  [unwired: 9 in, 1 out]
        n74 = Multiply(x=20 ("y"), y=w261) -> (x*y=w246:dbl)
        n75 = Unbundle(w239) -> ("tdms file out"=w238:refnum<k34>, "tdms file out"=w237:refnum<k34>, "tdms file out"=w236:refnum<k34>, "tdms file out"=w235:refnum<k34>)
        n76 = Unbundle(w224) -> ("Use Channel 0"=w223:bool, "Use Channel 1"=w222:bool, "Use Channel 2"=w221:bool, "Use Channel 3"=w220:bool)
        n77 = case shown="True" w220 {
          tunnel: w245 -> [_ w276]
          tunnel: [refnum<k34> refnum ("tdms file out") w274] -> w215
          tunnel: w238 -> [_ w272]
          frame False {
          }
          frame True {
            n78 = Index Array(array=w276, index (row)=3 ("index")) -> (element=w275:dbl[])  [unwired: 1 in]
            n79 = TDMS Write(0:w272, 7:string[] ["Channel 3"] ("channel name(s) in (Untitled)"), 9:w275) -> (4:w274:refnum<k34>)  [unwired: 3 in, 3 out]
          }
        }
        n80 = case shown="True" w221 {
          tunnel: w245 -> [_ w283]
          tunnel: [refnum<k34> refnum ("tdms file out") w281] -> w212
          tunnel: w237 -> [_ w279]
          frame False {
          }
          frame True {
            n81 = Index Array(array=w283, index (row)=2 ("index")) -> (element=w282:dbl[])  [unwired: 1 in]
            n82 = TDMS Write(0:w279, 7:string[] ["Channel 2"] ("channel name(s) in (Untitled)"), 9:w282) -> (4:w281:refnum<k34>)  [unwired: 3 in, 3 out]
          }
        }
        n83 = case shown="True" w222 {
          tunnel: w245 -> [_ w290]
          tunnel: [refnum<k34> refnum ("tdms file out") w289] -> w214
          tunnel: w236 -> [_ w286]
          frame False {
          }
          frame True {
            n84 = Index Array(array=w290, index (row)=1 ("index")) -> (element=w288:dbl[])  [unwired: 1 in]
            n85 = TDMS Write(0:w286, 7:string[] ["Channel 1"] ("channel name(s) in (Untitled)"), 9:w288) -> (4:w289:refnum<k34>)  [unwired: 3 in, 3 out]
          }
        }
        n86 = case shown="True" w223 {
          tunnel: w245 -> [_ w297]
          tunnel: [refnum<k34> refnum ("tdms file out") w295] -> w213
          tunnel: w235 -> [_ w293]
          frame False {
          }
          frame True {
            n87 = Index Array(array=w297, index (row)=0 ("index")) -> (element=w296:dbl[])  [unwired: 1 in]
            n88 = TDMS Write(0:w293, 7:string[] ["Channel 4"] ("channel name(s) in (Untitled)"), 9:w296) -> (4:w295:refnum<k34>)  [unwired: 3 in, 3 out]
          }
        }
        n89 = case shown="True" w263 {
          tunnel: [Enum_State_Typedef."Record" ("State") Enum_State_Typedef."Stop" ("State")] -> w264
          frame False {
            # "Continue recording"
          }
          frame True {
            # "Finished recording"
            n90 = One Button Dialog(message="Recording is Finished") -> ()  [unwired: 1 in, 1 out]
          }
        }
        n91 = Bundle("data"=w245, w247, 0, 20, w246, "Use Channel 0"=w223) -> (w219:T10)  [unwired: 1 in]
        n92 = Bundle("data"=w245, w247, 1, w253, w246, "Use Channel 1"=w222) -> (w218:T11)  [unwired: 1 in]
        n93 = Bundle("data"=w245, w247, 2, w253, w246, "Use Channel 2"=w221) -> (w217:T12)  [unwired: 1 in]
        n94 = Bundle("data"=w245, w247, 3, w253, w246, "Use Channel 3"=w220) -> (w216:T13)  [unwired: 1 in]
        n95 = call "Waveform Generation.vi"("Cluster"=w219) -> ("Output Y Values"=w244:dbl[], "Waveform"=w229:waveform(dbl))  [unwired: 9 in]
        n96 = call "Waveform Generation.vi"("Cluster"=w218) -> ("Output Y Values"=w243:dbl[], "Waveform"=w228:waveform(dbl))  [unwired: 9 in]
        n97 = call "Waveform Generation.vi"("Cluster"=w217) -> ("Output Y Values"=w242:dbl[], "Waveform"=w227:waveform(dbl))  [unwired: 9 in]
        n98 = call "Waveform Generation.vi"("Cluster"=w216) -> ("Output Y Values"=w241:dbl[], "Waveform"=w226:waveform(dbl))  [unwired: 9 in]
        n99 = Build Array(w244, w243, w242, w241) -> (w240:dbl[][])
        n100 = Bundle("Waveform"=w229, "Waveform"=w228, "Waveform"=w227, "Waveform"=w226) -> (w234:T14)  [unwired: 1 in]
        n101 = Build Array(w229, w228, w227, w226) -> (w225:waveform(dbl)[])
        n102 = Bundle("tdms file out"=w215, "tdms file out"=w212, "tdms file out"=w214, "tdms file out"=w213) -> (w211:T7)  [unwired: 1 in]
        n103 = Unbundle(w234) -> ("Waveform"=w233:waveform(dbl), "Waveform"=w232:waveform(dbl), "Waveform"=w231:waveform(dbl), "Waveform"=w230:waveform(dbl))
        n104 = Unbundle(w211) -> ("tdms file out"=w210:refnum<k34>, "tdms file out"=w209:refnum<k34>, "tdms file out"=w208:refnum<k34>, "tdms file out"=w207:refnum<k34>)
      }
      frame "Clear Display" {
        w309 = waveform(dbl) {"t0"=timestamp(0 s since 1904-01-01), "dt"=1.0, "Y"=[]} ("Waveform")
        w310 = waveform(dbl)[] [] ("History Data")
        # "clears the data"
        # "Clears the graph"
        # "Clears the chart history"
        # "This clears the chart display"
        n105 = property on="Channel 0 Chart" class="WFChart (strict)"("History Data"=w310) -> ()  [unwired: 2 in, 2 out]
        n106 = property on="Channel 2 Chart" class="WFChart (strict)"("History Data"=w310) -> ()  [unwired: 2 in, 2 out]
        n107 = property on="Channel 1 Chart" class="WFChart (strict)"("History Data"=w310) -> ()  [unwired: 2 in, 2 out]
        n108 = property on="Channel 3 Chart" class="WFChart (strict)"("History Data"=w310) -> ()  [unwired: 2 in, 2 out]
        n109 = property on="Overview Chart" class="WFChart (strict)"("History Data"=waveform(dbl)[][] []) -> ()  [unwired: 2 in, 2 out]
        n110 = Unbundle(w306) -> ("tdms file out"=w305:refnum<k34>, "tdms file out"=w304:refnum<k34>, "tdms file out"=w303:refnum<k34>, "tdms file out"=w302:refnum<k34>)
      }
      frame "Preview Data" {
        # "Turns off the X auto scale"
        n111 = property on="Channel 0 Chart" class="WFChart (strict)"("XScale.ScaleFit"=u8 0 ("X Scale.Scale Fit")) -> ()  [unwired: 2 in, 2 out]
        n112 = property on="Channel 2 Chart" class="WFChart (strict)"("XScale.ScaleFit"=u8 0 ("X Scale.Scale Fit")) -> ()  [unwired: 2 in, 2 out]
        n113 = property on="Overview Chart" class="WFChart (strict)"("XScale.ScaleFit"=u8 0 ("X Scale.Scale Fit")) -> ()  [unwired: 2 in, 2 out]
        n114 = property on="Channel 3 Chart" class="WFChart (strict)"("XScale.ScaleFit"=u8 0 ("X Scale.Scale Fit")) -> ()  [unwired: 2 in, 2 out]
        n115 = property on="Channel 1 Chart" class="WFChart (strict)"("XScale.ScaleFit"=u8 0 ("X Scale.Scale Fit")) -> ()  [unwired: 2 in, 2 out]
        n116 = property on="Overview Chart" class="WFChart (strict)"("XScale.Maximum"=w339) -> ()  [unwired: 2 in, 2 out]
        n117 = property on="Channel 0 Chart" class="WFChart (strict)"("XScale.Maximum"=w339) -> ()  [unwired: 2 in, 2 out]
        n118 = property on="Channel 1 Chart" class="WFChart (strict)"("XScale.Maximum"=w339) -> ()  [unwired: 2 in, 2 out]
        n119 = property on="Channel 2 Chart" class="WFChart (strict)"("XScale.Maximum"=w339) -> ()  [unwired: 2 in, 2 out]
        n120 = property on="Channel 3 Chart" class="WFChart (strict)"("XScale.Maximum"=w339) -> ()  [unwired: 2 in, 2 out]
        n121 = Reciprocal(x=w355) -> (1/x=w365:dbl)
        n122 = Index Array(array=w338, index (row)=0) -> (element=w357:dbl[])  [unwired: 1 in]
        n123 = Divide(x=w355, y=10) -> (x/y=w366:dbl)
        n124 = Array Size(array=w357) -> (size(s)=w362:i32)
        n125 = Multiply(x=20 ("y"), y=w365) -> (x*y=w354:dbl)
        n126 = Multiply(x=w362, y=w354) -> (x*y=w361:dbl)
        n127 = call-poly <vilib>:"DAQmxBase Read.vi"("task/channels in"=w359, "number of samples per channel"=w366, "timeout"=100.0, "error in"=w358) -> ("data"=w342:dbl[][])  [unwired: 9 in, 2 out]
        n128 = Unbundle(w322) -> ("Use Channel 0"=w321:bool, "Use Channel 1"=w320:bool, "Use Channel 2"=w319:bool, "Use Channel 3"=w318:bool)
        n129 = call "Preview Waveform.vi"("Decimation Multiple"=u16 20, "Channel #"=i8 0, "In Use?"=w321, "New Y Values"=w342, "Old Y Values"=w338) -> ("Output Y Values"=w332:dbl[])  [unwired: 6 in]
        n130 = call "Preview Waveform.vi"("Decimation Multiple"=u16 20, "Channel #"=i8 1, "In Use?"=w320, "New Y Values"=w342, "Old Y Values"=w338) -> ("Output Y Values"=w331:dbl[])  [unwired: 6 in]
        n131 = call "Preview Waveform.vi"("Decimation Multiple"=u16 20, "Channel #"=i8 2, "In Use?"=w319, "New Y Values"=w342, "Old Y Values"=w338) -> ("Output Y Values"=w330:dbl[])  [unwired: 6 in]
        n132 = call "Preview Waveform.vi"("Decimation Multiple"=u16 20, "Channel #"=i8 3, "In Use?"=w318, "New Y Values"=w342, "Old Y Values"=w338) -> ("Output Y Values"=w329:dbl[])  [unwired: 6 in]
        n133 = Build Array(w332, w331, w330, w329) -> (w328:dbl[][])
        n134 = Bundle By Name("Y"=w332, "dt"=w354) -> (w337:waveform(dbl))  [unwired: 1 in]
        n135 = Bundle By Name("Y"=w331, "dt"=w354) -> (w336:waveform(dbl))  [unwired: 1 in]
        n136 = Bundle By Name("Y"=w330, "dt"=w354) -> (w335:waveform(dbl))  [unwired: 1 in]
        n137 = Bundle By Name("Y"=w329, "dt"=w354) -> (w334:waveform(dbl))  [unwired: 1 in]
        n138 = Less?(x=w361, y=w339) -> (x < y?=w356:bool)
        n139 = Build Array(w337, w336, w335, w334) -> (w333:waveform(dbl)[])
        n140 = case shown="False" w356 {
          tunnel: [Enum_State_Typedef."Prepreview Handling" ("State") Enum_State_Typedef."Preview Data" ("State")] -> w363
          frame False {
          }
          frame True {
          }
        }
        n141 = Unbundle(w327) -> ("tdms file out"=w326:refnum<k34>, "tdms file out"=w325:refnum<k34>, "tdms file out"=w324:refnum<k34>, "tdms file out"=w323:refnum<k34>)
      }
      frame "Open FIle" {
        w381 = refnum<k34> refnum ("tdms file out")
        w382 = waveform(dbl) {"t0"=timestamp(0 s since 1904-01-01), "dt"=1.0, "Y"=[]} ("Waveform")
        n142 = call "File Dialog5"() -> ("selected path"=w383:path)  [unwired: 12 in, 3 out]
        n143 = call <vilib>:"TDMS - File Viewer.vi"("file path"=w383) -> ("error out"=w379:errorcluster)  [unwired: 5 in, 1 out]
      }
      frame "Create File" {
        # "This Creates and writes the header of the file with all the user inputted data"
        n144 = Get Date/Time String(date format (0)=enum16{"short", "long", "abbreviated"}."short") -> (date string=→"Date mm/dd/yy":string, time string=→"Start Time hr/min":string)  [unwired: 2 in]
        n145 = Unbundle(w388) -> ("Use Channel 0"=w387:bool, "Use Channel 1"=w386:bool, "Use Channel 2"=w385:bool, "Use Channel 3"=w384:bool)
        n146 = Enqueue Element(queue=w411, element=Enum_State_Typedef."Record", error in (no error)=w410) -> ()  [unwired: 1 in, 3 out]
        n147 = case shown="True" w385 {
          tunnel: [refnum<k34> refnum ("tdms file out") w429] -> w397
          frame False {
          }
          frame True {
            n148 = call "File Dialog2"("prompt"="Select or Create a File for Channel 2") -> ("selected path"=w434:path)  [unwired: 11 in, 3 out]
            n149 = TDMS Open(10:T5."create" ("operation (0:open)"), 11:w434) -> (3:w432:refnum<k34>)  [unwired: 5 in, 1 out]
            n150 = call "Header Data Creator.vi"("tdms file in"=w432, "Amplifier Metadata"="Amplifier Channel 1", "User Data"="User Data Channel 1") -> ("tdms file out"=w429:refnum<k34>)  [unwired: 6 in, 1 out]
          }
        }
        n151 = case shown="True" w387 {
          tunnel: [refnum<k34> refnum ("tdms file out") w415] -> w395
          frame False {
          }
          frame True {
            n152 = call "File Dialog4"("prompt"="Select or Create a File for Channel 0") -> ("selected path"=w418:path)  [unwired: 11 in, 3 out]
            n153 = TDMS Open(10:T5."create" ("operation (0:open)"), 11:w418) -> (3:w416:refnum<k34>)  [unwired: 5 in, 1 out]
            n154 = call "Header Data Creator.vi"("tdms file in"=w416, "Amplifier Metadata"="Amplifier Channel 3", "User Data"="User Data Channel 3") -> ("tdms file out"=w415:refnum<k34>)  [unwired: 6 in, 1 out]
          }
        }
        n155 = case shown="True" w384 {
          tunnel: [refnum<k34> refnum ("tdms file out") w439] -> w398
          frame False {
          }
          frame True {
            n156 = call "File Dialog"("prompt"="Select or Create a File for Channel 3") -> ("selected path"=w443:path)  [unwired: 11 in, 3 out]
            n157 = TDMS Open(10:T5."create" ("operation (0:open)"), 11:w443) -> (3:w440:refnum<k34>)  [unwired: 5 in, 1 out]
            n158 = call "Header Data Creator.vi"("tdms file in"=w440, "Amplifier Metadata"="Amplifier Channel 0", "User Data"="User Data Channel 0") -> ("tdms file out"=w439:refnum<k34>)  [unwired: 6 in, 1 out]
          }
        }
        n159 = case shown="True" w386 {
          tunnel: [refnum<k34> refnum ("tdms file out") w421] -> w396
          frame False {
          }
          frame True {
            n160 = call "File Dialog3"("prompt"="Select or Create a File for Channel 1") -> ("selected path"=w426:path)  [unwired: 11 in, 3 out]
            n161 = TDMS Open(10:T5."create" ("operation (0:open)"), 11:w426) -> (3:w422:refnum<k34>)  [unwired: 5 in, 1 out]
            n162 = call "Header Data Creator.vi"("tdms file in"=w422, "Amplifier Metadata"="Amplifier Channel 2", "User Data"="User Data Channel 2") -> ("tdms file out"=w421:refnum<k34>)  [unwired: 6 in, 1 out]
          }
        }
        n163 = Unbundle(w393) -> ("Waveform"=w392:waveform(dbl), "Waveform"=w391:waveform(dbl), "Waveform"=w390:waveform(dbl), "Waveform"=w389:waveform(dbl))  [unwired: 1 out]
      }
      frame "Prepreview Handling" {
        w451 = waveform(dbl)[] [] ("History Data")
        w452 = waveform(dbl) {"t0"=timestamp(0 s since 1904-01-01), "dt"=1.0, "Y"=[]}
        # "This clears the Chart history"
        # "This clears the data before the preview data state starts"
        n164 = property on="Channel 2 Chart" class="WFChart (strict)"("History Data"=w451) -> ()  [unwired: 2 in, 2 out]
        n165 = property on="Channel 3 Chart" class="WFChart (strict)"("History Data"=w451) -> ()  [unwired: 2 in, 2 out]
        n166 = property on="Channel 1 Chart" class="WFChart (strict)"("History Data"=w451) -> ()  [unwired: 2 in, 2 out]
        n167 = property on="Channel 0 Chart" class="WFChart (strict)"("History Data"=w451) -> ()  [unwired: 2 in, 2 out]
        n168 = property on="Overview Chart" class="WFChart (strict)"("History Data"=waveform(dbl)[][] []) -> ()  [unwired: 2 in, 2 out]
        n169 = Unbundle(w448) -> ("tdms file out"=w447:refnum<k34>, "tdms file out"=w446:refnum<k34>, "tdms file out"=w445:refnum<k34>, "tdms file out"=w444:refnum<k34>)
      }
    }
    "Channel 0 Chart" <- w34
    "State" <- w47
    "Channel 1 Chart" <- w32
    "Channel 3 Chart" <- w33
    "Channel 2 Chart" <- w31
    "Overview Chart" <- w26
  }
  n170 = while {
    tunnel: w8 -> [w464]
    tunnel: w7 -> [w463]
    tunnel: w2 -> [w461]
    tunnel: w1 -> [w460]
    stop <- w462 stop-if-true
    # "Event Handling Loop"
    n171 = event shown="[8] \"Clear Display\": Value Change" {
      selector: _ -> [_ _ _ _ _ _ _ _ _]
      dyn-events: _ -> [_ _ _ _ _ _ _ _ _]
      timeout: _ -> [_ _ _ _ _ _ _ _ _]
      tunnel: [FALSE ("Exit Button") "Exit Button" FALSE ("Exit Button") FALSE ("Exit Button") FALSE ("Exit Button") FALSE ("Exit Button") FALSE ("Exit Button") FALSE ("Exit Button") FALSE ("Exit Button")] -> w462
      tunnel: w464 -> [_ w470 w477 w481 w487 w491 w497 w503 w507]
      tunnel: w463 -> [_ w469 w476 w480 w486 w490 w496 w502 w506]
      tunnel: [_ w468 w474 _ w484 _ w494 w500 _] -> _
      tunnel: [_ w467 w473 _ w483 _ w495 w501 _] -> _
      event Timeout {
        n172 = event-data() -> ()  [unwired: 1 in, 3 out]
      }
      event "Exit Button": Value Change {
        n173 = event-data() -> ()  [unwired: 1 in, 1 out]
        n174 = Enqueue Element(queue=w470, element=Enum_State_Typedef."Exit", error in (no error)=w469) -> (queue out=w468:refnum<queue>, error out=w467:errorcluster)  [unwired: 1 in, 1 out]
      }
      event "Preview Button": Value Change {
        n175 = event-data() -> ()  [unwired: 1 in, 6 out]
        n176 = Enqueue Element(queue=w477, element=Enum_State_Typedef."Preview Data", error in (no error)=w476) -> (queue out=w474:refnum<queue>, error out=w473:errorcluster)  [unwired: 1 in, 1 out]
      }
      event "Stop Preview": Value Change {
        n177 = event-data() -> ()  [unwired: 1 in, 6 out]
        n178 = Enqueue Element(queue=w481, element=Enum_State_Typedef."", error in (no error)=w480) -> ()  [unwired: 1 in, 3 out]
      }
      event "Open Button": Value Change {
        n179 = event-data() -> ()  [unwired: 1 in, 6 out]
        n180 = Enqueue Element(queue=w487, element=Enum_State_Typedef."Open FIle", error in (no error)=w486) -> (queue out=w484:refnum<queue>, error out=w483:errorcluster)  [unwired: 1 in, 1 out]
      }
      event "OK Button": Value Change {
        n181 = event-data() -> ()  [unwired: 1 in, 6 out]
        n182 = Enqueue Element(queue=w491, element=Enum_State_Typedef."Set the Sample Clock", error in (no error)=w490) -> ()  [unwired: 1 in, 3 out]
      }
      event "Stop Button": Value Change {
        n183 = event-data() -> ()  [unwired: 1 in, 6 out]
        n184 = Enqueue Element(queue=w497, element=Enum_State_Typedef."Stop", error in (no error)=w496) -> (queue out=w494:refnum<queue>, error out=w495:errorcluster)  [unwired: 1 in, 1 out]
      }
      event "Record Button": Value Change {
        n185 = event-data() -> ()  [unwired: 1 in, 6 out]
        n186 = Enqueue Element(queue=w503, element=Enum_State_Typedef."Create File", error in (no error)=w502) -> (queue out=w500:refnum<queue>, error out=w501:errorcluster)  [unwired: 1 in, 1 out]
      }
      event "Clear Display": Value Change {
        n187 = event-data() -> ()  [unwired: 1 in, 6 out]
        n188 = Enqueue Element(queue=w507, element=Enum_State_Typedef."Clear Display", error in (no error)=w506) -> ()  [unwired: 1 in, 3 out]
      }
    }
    n189 = Enqueue Element(queue=w461, element=w462, error in (no error)=w460) -> ()  [unwired: 1 in, 3 out]
  }
